vi "SendCmd.vi"(11 "Function":T1(ring)) -> (3 "concatenated string":string)   [LabVIEW 2018]
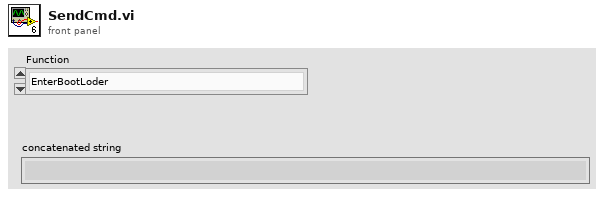
[diagram p1: front panel]
types:
  T1 = enum16{"EnterBootLoder", "StartToUpdate", "JumpToApp"}
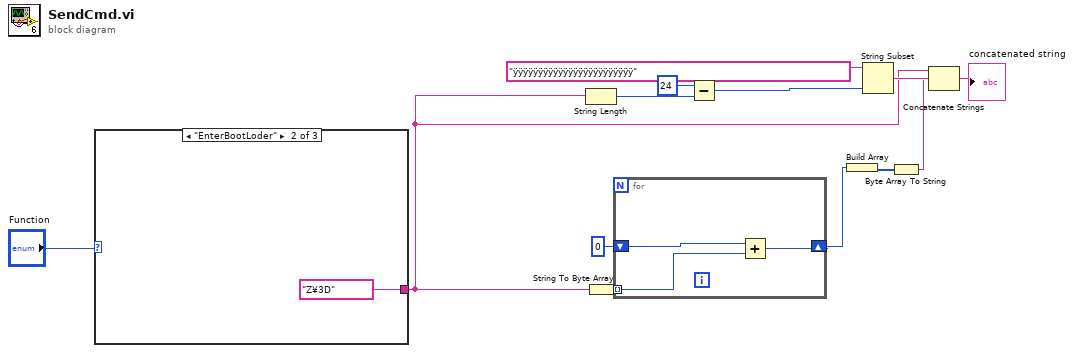
[diagram p0: block diagram]
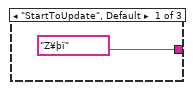
[diagram p2: hidden frame]
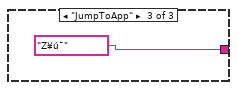
[diagram p3: hidden frame]
diagram:
  n1 = case shown="\"EnterBootLoder\"" "Function" {
    tunnel: ["Z¥þï" ("string") "Z¥3D" ("string") "Z¥ú¯" ("string")] -> w2
    frame "StartToUpdate", Default {
    }
    frame "EnterBootLoder" {
    }
    frame "JumpToApp" {
    }
  }
  n2 = String Length(string=w2) -> (length=w11:i32)
  n3 = String To Byte Array(string=w2) -> (unsigned byte array=w13:u8[])
  n4 = for {
    shift-right: [w18] -> w7
    shift-left: u8 0 -> [w19]
    tunnel: w13 -> [w17] mode=indexing
    n5 = Add(x=w19, y=w17) -> (x+y=w18:u8)
  }
  n6 = Subtract(x=24, y=w11) -> (x-y=w8:i32)
  n7 = Build Array(w7) -> (w6:u8[])
  n8 = String Subset(string="ÿÿÿÿÿÿÿÿÿÿÿÿÿÿÿÿÿÿÿÿÿÿÿÿ", length (rest)=w8) -> (substring=w5:string)  [unwired: 1 in]
  n9 = Byte Array To String(unsigned byte array=w6) -> (string=w4:string)
  n10 = Concatenate Strings(w2, w4, w5) -> (→"concatenated string":string)
